vi "Scan Engine and FPGA User Variables Host Demo.vi"() -> ()   [LabVIEW 2025]
uses:
  FPGA IP/Types/PWM.Measure.Digital.Result.ctl
  FPGA IP/Types/PWM.Generate.Digital.Convert.Settings.ctl
  FPGA IP/Types/PWM.Measure.Digital.Measurement.ctl
  <vilib>/Platform/TimedLoop/XDataNode/timing_clust.ctl
  <vilib>/Platform/TimedLoop/XDataNode/nitl_modes.ctl
  <vilib>/Platform/TimedLoop/XDataNode/wakeup.ctl
  <vilib>/Platform/TimedLoop/XDataNode/loadnilvce.vi
  <vilib>/FPGAPlugInAG/cRIO-9045/niLvFpga_Open_cRIO-9045.vi
  <vilib>/rvi/interface/common/dynamic/niFpgaDynamicAddResources.vi
  <vilib>/FPGAPlugInAG/Dynamic/niLvFpga_Close_Dynamic.vi
  <vilib>/platform/TimedLoop/XDataNode/XDataNode.xnode
  <vilib>/rvi/interface/nirviOpenFPGA/nirviOpenFPGA.xnode
  FPGA Bitfiles/scanengineexampl_FPGATarget_ExampleFPGA_9nPm7+spJUY.lvbitx
  <vilib>/rvi/interface/nirviCloseFPGA/nirviCloseFPGA.xnode
  <resource>/objmgr/cRIO.rc
  FPGA IP/Speciality FPGA IO.lvlib
  <vilib>/Platform/TimedLoop/XDataNode/XDNodeRunTimeDep.lvlib
panel:
  in  "stop control":bool
  out "AI0":dbl
  in  "AO0":dbl
  in  "PWM Generation Settings":T1={"ACTIVE EDGE"=TRUE, "FREQ"=5.0, "DC"=48.0}
  out "PWM Result":T2
  in  "stop acq":bool
  out "Bulk Data":dbl[](array[numeric])
  out "error out":errorcluster
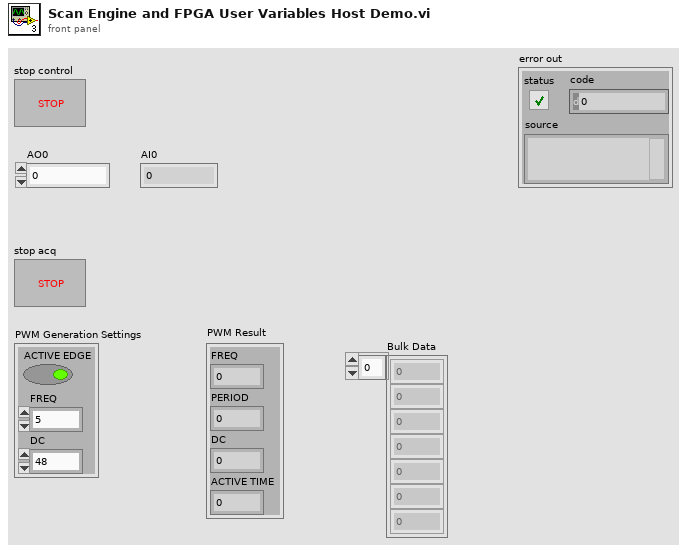
[diagram p1: front panel]
types:
  T1 = typedef "Speciality FPGA IO.lvlib/PWM.Generate.Digital.Convert.Settings.ctl" = cluster{"ACTIVE EDGE":bool, "FREQ":sgl, "DC":sgl}
  T2 = typedef "Speciality FPGA IO.lvlib/PWM.Measure.Digital.Result.ctl" = cluster{"FREQ":sgl, "PERIOD":sgl, "DC":sgl, "ACTIVE TIME":sgl}
  T3 = typedef "Speciality FPGA IO.lvlib/PWM.Measure.Digital.Measurement.ctl" = cluster{"ACTIVE TICKS":u32, "INACTIVE TICKS":u32, "ACQ TICKS":u32}
  T4 = typedef "Speciality FPGA IO.lvlib/PWM.Generate.Digital.Settings.ctl" = cluster{"ACTIVE EDGE":bool, "ACTIVE TICKS":u32, "INACTIVE TICKS":u32}
  T5 = typedef "XDNodeRunTimeDep.lvlib/timing_clust.ctl" = cluster{"Expected End [f-1]":u64, "Actual End [f-1]":u64, "Finished Late? [f-1]":bool, "Expected End [i-1]":u64, "Actual End [i-1]":u64, "Finished Late? [i-1]":bool, "Expected Start [i]":u64, "Actual Start [i]":u64, "Expected Start [f]":u64, "Actual Start [f]":u64, "Source Name":string, "Structure Name":string, "Period":i64, "Deadline":i64, "Offset":i64, "Start":i64, "Priority":i32, "Timeout":i32, "Mode":T6, "Wakeup Reason":T7, "Error":errorcluster, "Source Type":string, "Secondary Source Type":string, "Global End Time":u64, "Global Start Time":u64, "Frame Duration":u64, "Iteration Duration":u64, "Assigned CPU":i32, "I/O Scan Engine Mode":u32}
  T6 = typedef "XDNodeRunTimeDep.lvlib/nitl_modes.ctl" = enum32{"No Change", "Process missed periods, maintain original phase", "Discard missed periods, maintain original phase", "Process missed periods, ignore original phase", "Discard missed periods, ignore original phase"}
  T7 = typedef "XDNodeRunTimeDep.lvlib/wakeup.ctl" = enum32{"Normal", "Aborted", "Asynchronous wakeup", "Timing source error", "Timed loop error", "Timeout"}
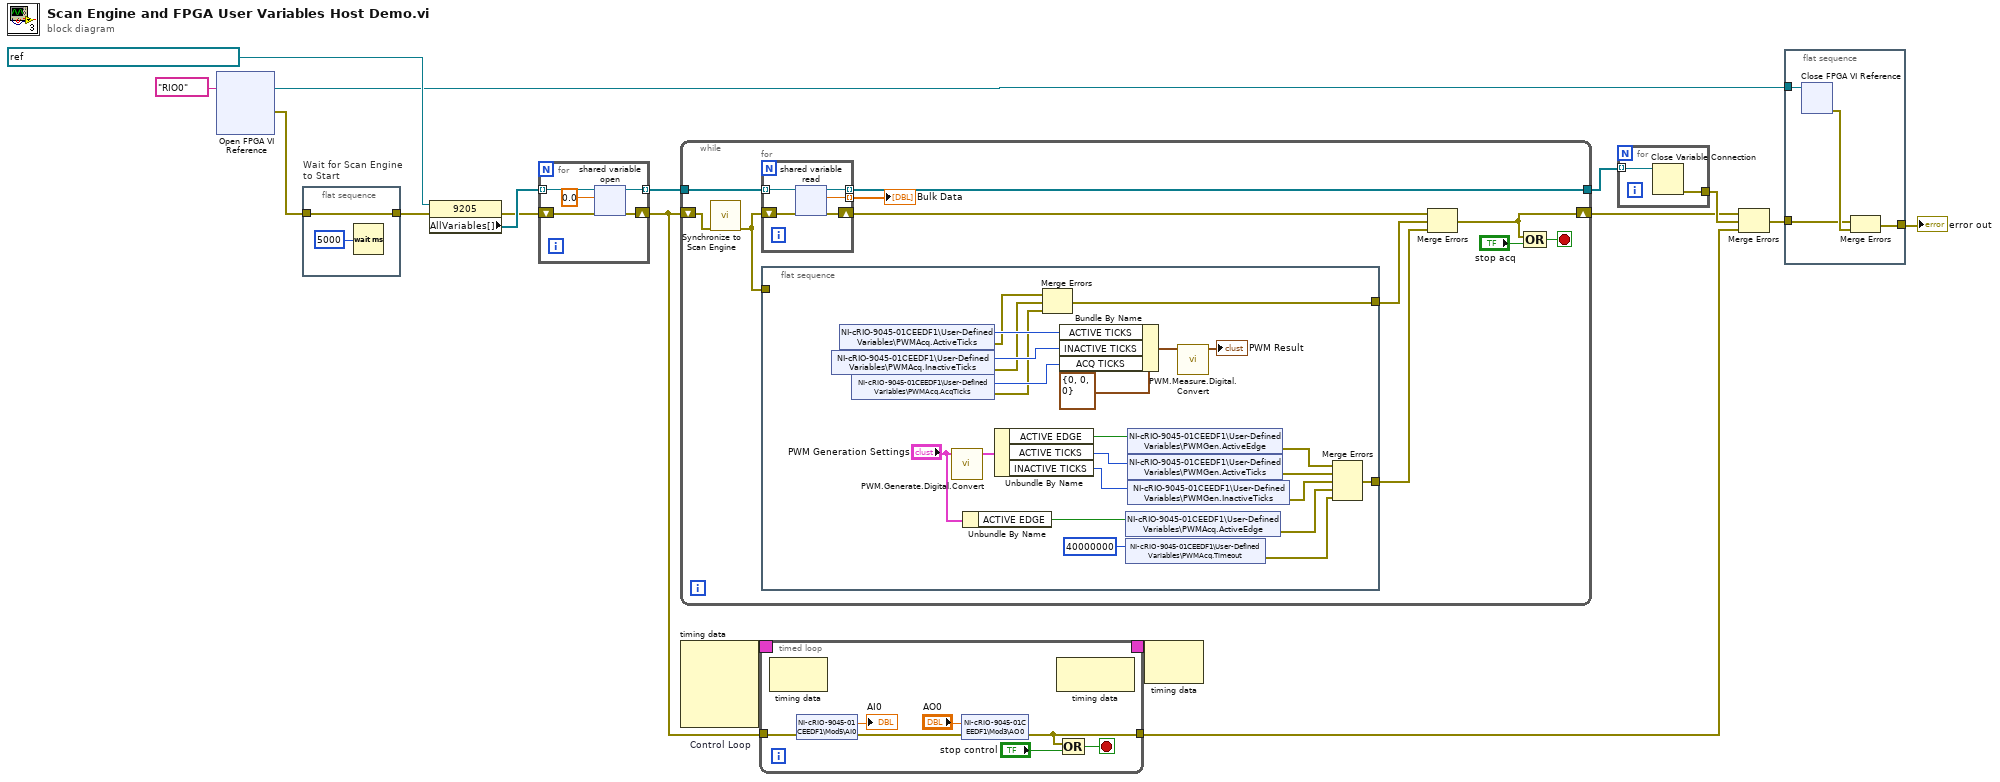
[diagram p0: block diagram]
diagram:
  n1 = xnode "Open FPGA VI Reference"("resource name"=tag "RIO0") -> ("FPGA VI Reference Out"=w6:refnum<k20>, "error out"=w1:errorcluster)  [unwired: 1 in]
  n2 = flat-sequence "Wait for Scan Engine\nto Start" {
    tunnel: [w19] -> w2
    tunnel: w1 -> [w19]
    frame #0 {
      n3 = Wait (ms)(milliseconds to wait=u32 5000) -> ()  [unwired: 1 out]
    }
  }
  n4 = property class="9205"(reference=refnum<k21> "ni.var.io://ni-crio-9045-01ceedf1/Mod4" ("9205 Refnum"), error in=w2) -> (error out=w14:errorcluster, "AllVariables[]"=w16:refnum<k21>[])  [unwired: 1 out]
  n5 = for {
    tunnel: w16 -> [w24] mode=indexing
    tunnel: [w22] -> w15 mode=indexing
    shift-right: [w21] -> w3
    shift-left: w14 -> [w20]
    n6 = shared-variable-open(w24, w20, 0.0) -> (w22:refnum<k21>, w21:errorcluster)  [unwired: 1 in]
  }
  n7 = while {
    tunnel: w15 -> [w35]
    shift-right: [w25] -> w11
    shift-left: w3 -> [w34]
    tunnel: [w30] -> w13
    stop <- w31 stop-if-true
    n8 = call <vilib>:"Synchronize to Scan Engine.vi"("error in (no error)"=w34) -> ("error out"=w29:errorcluster)  [unwired: 9 in, 1 out]
    n9 = for {
      tunnel: w35 -> [w63] mode=indexing
      tunnel: [w61] -> w33 mode=indexing
      shift-right: [w60] -> w26
      shift-left: w29 -> [w62]
      tunnel: [w59] -> w30 mode=indexing
      n10 = shared-variable-read(w63, w62) -> (w59:refnum<k21>, w60:errorcluster, w61:dbl)  [unwired: 1 out]
    }
    "Bulk Data" <- w33
    n11 = flat-sequence {
      tunnel: w29 -> [_]
      tunnel: [w37] -> w28
      tunnel: [w36] -> w27
      frame #0 {
        n12 = shared-variable "NI-cRIO-9045-01CEEDF1\\User-Defined Variables\\PWMAcq.InactiveTicks"() -> (w56:u32, error out=w44:errorcluster)  [unwired: 1 in]
        n13 = shared-variable "NI-cRIO-9045-01CEEDF1\\User-Defined Variables\\PWMAcq.ActiveTicks"() -> (w55:u32, error out=w45:errorcluster)  [unwired: 1 in]
        n14 = shared-variable "NI-cRIO-9045-01CEEDF1\\User-Defined Variables\\PWMAcq.AcqTicks"() -> (w57:u32, error out=w43:errorcluster)  [unwired: 1 in]
        n15 = call "PWM.Generate.Digital.Convert.vi"("Settings"="PWM Generation Settings") -> ("Settings"=w50:T4)  [unwired: 10 in]
        n16 = Unbundle By Name("PWM Generation Settings") -> ("ACTIVE EDGE"=w46:bool)
        n17 = Unbundle By Name(w50) -> ("ACTIVE EDGE"=w51:bool, "ACTIVE TICKS"=w52:u32, "INACTIVE TICKS"=w53:u32)
        n18 = Merge Errors(w45, w44, w43) -> (w37:errorcluster)
        n19 = Bundle By Name(cluster=T3 {"ACTIVE TICKS"=0, "INACTIVE TICKS"=0, "ACQ TICKS"=0} ("Measurement"), "ACTIVE TICKS"=w55, "INACTIVE TICKS"=w56, "ACQ TICKS"=w57) -> (w54:T3)
        n20 = shared-variable "NI-cRIO-9045-01CEEDF1\\User-Defined Variables\\PWMAcq.ActiveEdge"(w46) -> (error out=w39:errorcluster)  [unwired: 1 in]
        n21 = shared-variable "NI-cRIO-9045-01CEEDF1\\User-Defined Variables\\PWMAcq.Timeout"(u32 40000000 ("PWMAcq.Timeout")) -> (error out=w38:errorcluster)  [unwired: 1 in]
        n22 = shared-variable "NI-cRIO-9045-01CEEDF1\\User-Defined Variables\\PWMGen.ActiveEdge"(w51) -> (error out=w42:errorcluster)  [unwired: 1 in]
        n23 = shared-variable "NI-cRIO-9045-01CEEDF1\\User-Defined Variables\\PWMGen.ActiveTicks"(w52) -> (error out=w41:errorcluster)  [unwired: 1 in]
        n24 = shared-variable "NI-cRIO-9045-01CEEDF1\\User-Defined Variables\\PWMGen.InactiveTicks"(w53) -> (error out=w40:errorcluster)  [unwired: 1 in]
        n25 = call "PWM.Measure.Digital.Convert.vi"("Measurement"=w54) -> ("Result"=→"PWM Result":T2)  [unwired: 10 in]
        n26 = Merge Errors(w42, w41, w40, w39, w38) -> (w36:errorcluster)
      }
    }
    n27 = Merge Errors(w26, w28, w27) -> (w25:errorcluster)
    n28 = Compound Arithmetic op=OR(w25, "stop acq") -> (w31:bool)
  }
  n29 = node-c288 "Control Loop"() -> (w10:T5)  [unwired: 4 in]
  n30 = timed-loop {
    timing: w10 -> [_]
    timing-out: [_] -> w9
    tunnel: w3 -> [w68]
    tunnel: [w64] -> w7
    stop <- w65 stop-if-true
    n31 = node-c288() -> ()  [unwired: 1 in, 1 out]
    n32 = shared-variable "NI-cRIO-9045-01CEEDF1\\Mod5\\AI0"(error in=w68) -> (→"AI0":dbl, error out=w67:errorcluster)
    n33 = shared-variable "NI-cRIO-9045-01CEEDF1\\Mod3\\AO0"("AO0", error in=w67) -> (error out=w64:errorcluster)
    n34 = node-c288() -> ()  [unwired: 1 in, 1 out]
    n35 = Compound Arithmetic op=OR(w64, "stop control") -> (w65:bool)
  }
  n36 = node-c288(w9) -> ()  [unwired: 1 out]
  n37 = for {
    tunnel: w13 -> [w74] mode=indexing
    tunnel: [w73] -> w12
    n38 = Close Variable Connection(11:w74) -> (0:w73:errorcluster)  [unwired: 1 in]
  }
  n39 = Merge Errors(w11, w12, w7) -> (w5:errorcluster)
  n40 = flat-sequence {
    tunnel: w6 -> [w78]
    tunnel: w5 -> [w76]
    tunnel: [w75] -> w4
    frame #0 {
      n41 = xnode "Close FPGA VI Reference"("FPGA VI Reference In"=w78) -> ("error out"=w77:errorcluster)  [unwired: 1 in]
      n42 = Merge Errors(w76, w77) -> (w75:errorcluster)
    }
  }
  "error out" <- w4
